vi "parseTemperatureError.vi"(8 "error in (no error)":errorcluster, 10 "DynamicFrameParser":refnum<class "DynamicFrameParser.lvclass">, 11 "MTILC in":refnum<class "MTILC.lvclass">) -> (0 "error out":errorcluster, 3 "MTILC out":refnum<class "MTILC.lvclass">)   [LabVIEW 2016, in "RTMTILC.lvlib" / "MTILC.lvclass"]
uses:
  MTILC.lvclass
  Common_RT_Modbus/DynamicFrameParser/DynamicFrameParser.lvclass
  MTILC.lvclass/MTILC.ctl
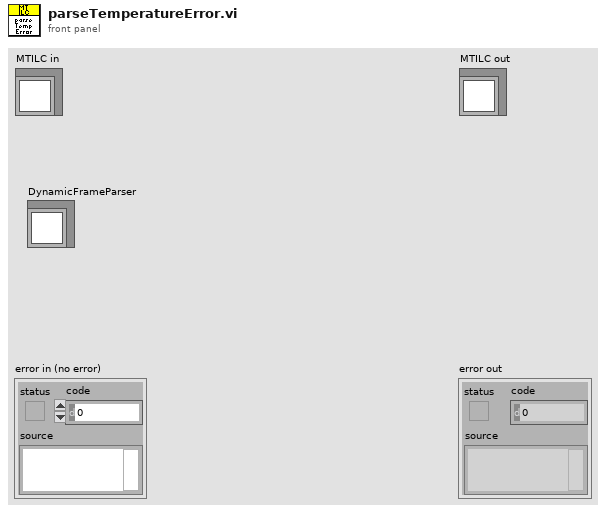
[diagram p1: front panel]
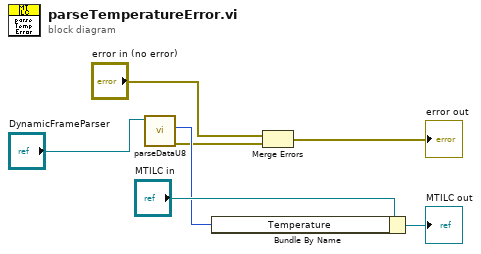
[diagram p0: block diagram]
diagram:
  n1 = call "parseDataU8.vi"("FrameParser in"="DynamicFrameParser") -> ("error out"=w1:errorcluster, "Data"=w2:u8)  [unwired: 8 in, 1 out]
  n2 = Bundle By Name(cluster="MTILC in", "Temperature"=w2) -> (→"MTILC out":refnum<class "MTILC.lvclass">)
  n3 = Merge Errors("error in (no error)", w1) -> (→"error out":errorcluster)
